vi "Read5160Record.vi"(11 "scope params":T1={"scope mode"=enum."Stopped", "ticker"=refnum, "record length"=0, "FPGA ref"=refnum, "P2P params"={"instrument handle"="", "stream session"=refnum, "scale"={"offset"=0.0, "gain"=0.0, "reserved 1"=0.0, "reserved 2"=0.0}, "actual sample rate"=10000000.0, "Trigger"=enum."PFI 0", "SCOPE Resource"="Dev1", "input impedance"=0}, "FPGA ref 5160"=refnum, "data mode"=enum."Real IO"} {"P2P params"."input impedance" items=["1 mega ohm"=0, "50 ohms"=2]; "P2P params"."actual sample rate" format="%.2p"}) -> (1 "Num elements":i32, 2 "data":i16[][](array[numeric]), 3 "scope params out":T1={"scope mode"=enum."Stopped", "ticker"=refnum, "record length"=0, "FPGA ref"=refnum, "P2P params"={"instrument handle"="", "stream session"=refnum, "scale"={"offset"=0.0, "gain"=0.0, "reserved 1"=0.0, "reserved 2"=0.0}, "actual sample rate"=10000000.0, "Trigger"=enum."PFI 0", "SCOPE Resource"="Dev1", "input impedance"=0}, "FPGA ref 5160"=refnum, "data mode"=enum."Real IO"} {"P2P params"."input impedance" items=["1 mega ohm"=0, "50 ohms"=2]; "P2P params"."actual sample rate" format="%.2p"}, 5 "P2P overflow":bool)   [LabVIEW 2013]
uses:
  controls/scope_params.ctl
  Utilities/Ticker/Ticker.lvclass
  controls/ScopeMode.ctl
  Config/FPGAref.ctl
  P2P params.ctl
  trigger_source.ctl
  Config/5160FPGAref.ctl
  FPGA/DataMode.ctl
  <vilib>/rvi/interface/common/niFpgaWaitOnOcc.vi
  <vilib>/Utility/error.llb/Error Cluster From Error Code.vi
  <vilib>/rvi/errors/niLvFpgaAdjustHostInterfaceError.vi
  <vilib>/rvi/interface/nirviReadWriteControl/nirviReadWriteControl.xnode
  <vilib>/rvi/interface/nirviMethod/nirviMethod.xnode
  <vilib>/FPGAPlugInAG/Dynamic/niLvFpga_ReadFifo_Dynamic.vi
  <vilib>/rvi/errors/niLvFpgaMergeErrorWithErrorCode.vi
  <resource>/objmgr/PeerToPeerStream.rc
  NiFpgaLv.dll
  <vilib>/rvi/interface/Simulation/niFpgaSimulationCallBeginRW.vi
panel:
  out "Data":u64[](array[numeric])
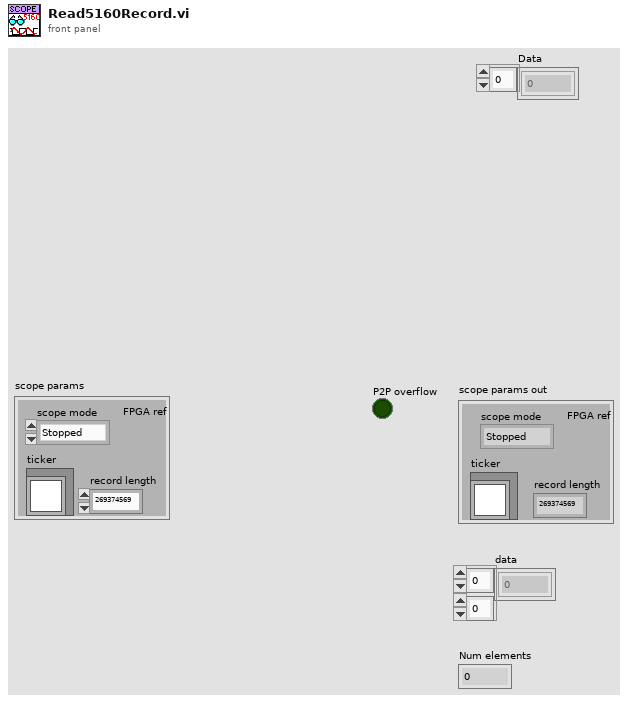
[diagram p1: front panel]
types:
  T1 = typedef "scope_params.ctl" = cluster{"scope mode":T2, "ticker":refnum<class "Ticker.lvclass">, "record length":u32, "FPGA ref":T3, "P2P params":T4, "FPGA ref 5160":T6, "data mode":T7}
  T2 = typedef "ScopeMode.ctl" = enum16{"Stopped", "Single", "Running"}
  T3 = typedef "FPGAref.ctl" = refnum<k20>
  T4 = typedef "P2P params.ctl" = cluster{"instrument handle":refnum<k15>, "stream session":refnum<k20>, "scale":cluster{"offset":dbl, "gain":dbl, "reserved 1":dbl, "reserved 2":dbl}, "actual sample rate":dbl, "Trigger":T5, "SCOPE Resource":refnum<k15>, "input impedance":u32}
  T5 = typedef "trigger_source.ctl" = enum16{"PFI 0", "PFI 1", "Software"}
  T6 = typedef "5160FPGAref.ctl" = refnum<k20>
  T7 = typedef "DataMode.ctl" = enum16{"Real IO", "Simulated"}
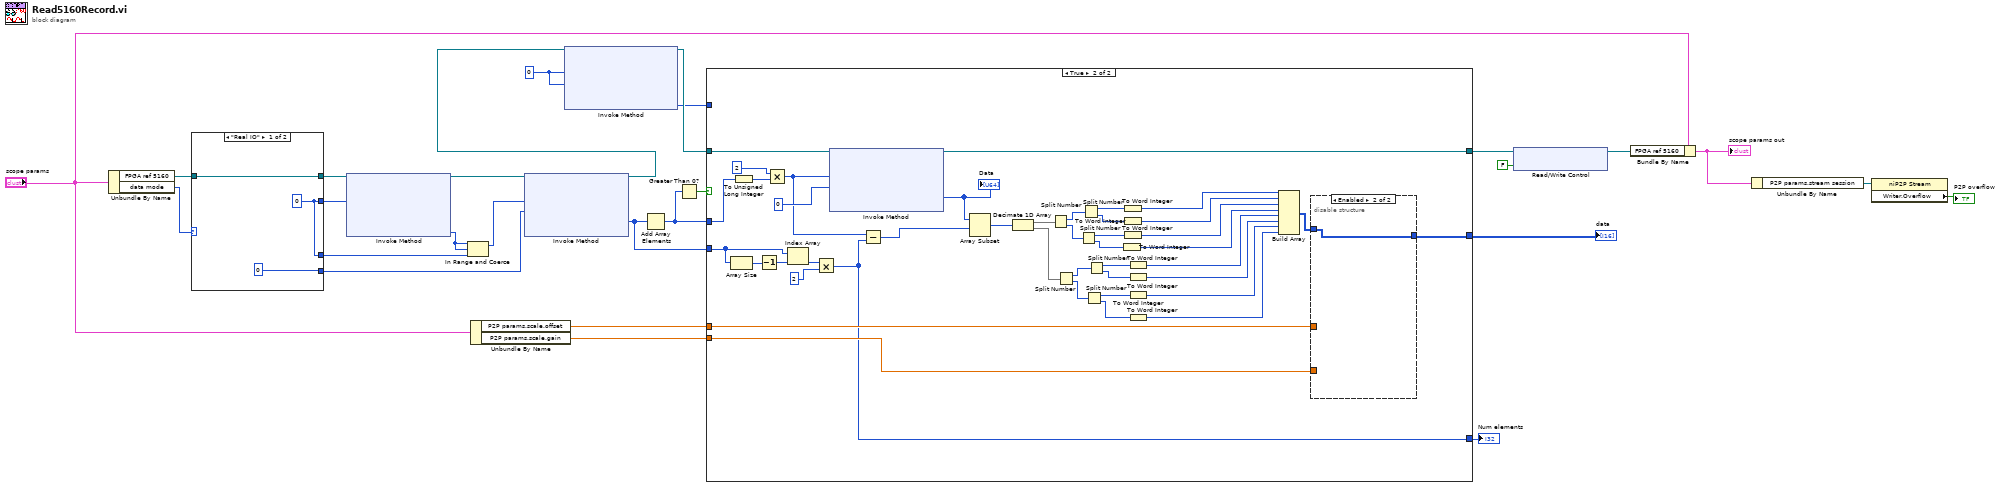
[diagram p0: block diagram]
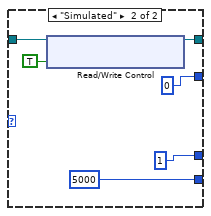
[diagram p2: hidden frame]
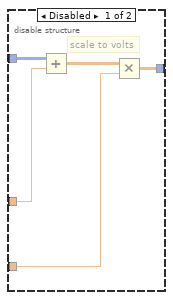
[diagram p4: hidden frame]
diagram:
  w7 = u32 0 ("Number of Elements")
  n1 = Unbundle By Name("scope params") -> ("FPGA ref 5160"=w14:T6, "data mode"=w15:T7)
  n2 = case shown="\"Real IO\"" w15 {
    tunnel: [0 ("Timeout (ms)") 5000 ("Timeout (ms)")] -> w4
    tunnel: w14 -> [w30 w36]
    tunnel: [w30 w34] -> w13
    tunnel: [w28 u32 0 ("Number of Elements")] -> w5
    tunnel: [w28 u32 1 ("Number of Elements")] -> w2
    frame "Real IO" {
      w28 = u32 0 ("Number of Elements")
    }
    frame "Simulated" {
      n3 = xnode "Read/Write Control"("FPGA VI Reference In"=w36, "Trigger simulated data"=TRUE) -> ("FPGA VI Reference Out"=w34:T6)  [unwired: 1 in, 1 out]
    }
  }
  n4 = xnode "Invoke Method"("FPGA VI Reference In"=w13, "Number of Elements"=w5) -> ("FPGA VI Reference Out"=w24:T6, "Elements Remaining"=w1:u32)  [unwired: 2 in, 2 out]
  n5 = In Range and Coerce(upper limit=w1, x=w1, lower limit=w2) -> (coerced(x)=w3:u32)  [unwired: 1 out]
  n6 = Unbundle By Name("scope params") -> ("P2P params.scale.offset"=w26:dbl, "P2P params.scale.gain"=w25:dbl)
  n7 = xnode "Invoke Method"("FPGA VI Reference In"=w24, "Number of Elements"=w3, "Timeout (ms)"=w4) -> ("FPGA VI Reference Out"=w9:T6, "Data"=w22:i32[])  [unwired: 1 in, 2 out]
  n8 = xnode "Invoke Method"("FPGA VI Reference In"=w9, "Number of Elements"=w7, "Timeout (ms)"=w7) -> ("FPGA VI Reference Out"=w8:T6, "Elements Remaining"=w6:u32)  [unwired: 1 in, 2 out]
  n9 = Add Array Elements(numeric array=w22) -> (sum=w23:i32)
  n10 = Greater Than 0?(x=w23) -> (x > 0?=w21:bool)
  n11 = case shown="True" w21 {
    tunnel: [_ w79] -> w27
    tunnel: w26 -> [_ w78]
    tunnel: w25 -> [_ w77]
    tunnel: w8 -> [w37 w53]
    tunnel: w23 -> [_ w45]
    tunnel: w22 -> [_ w52]
    tunnel: [w37 w51] -> w12
    tunnel: [_ w39] -> w20
    tunnel: w6 -> [_ _]
    frame False {
    }
    frame True {
      n12 = Array Size(array=w52) -> (size(s)=w49:i32)
      n13 = To Unsigned Long Integer(number=w45) -> (unsigned 32bit integer=w43:u32)
      n14 = Decrement(x=w49) -> (x-1=w48:i32)
      n15 = Multiply(x=u32 2, y=w43) -> (x*y=w38:u32)
      n16 = Index Array(array=w52, index=w48) -> (element=w41:i32)
      n17 = Multiply(x=w41, y=u32 2 ("x")) -> (x*y=w39:u32)
      n18 = xnode "Invoke Method"("FPGA VI Reference In"=w53, "Number of Elements"=w38, "Timeout (ms)"=0) -> ("FPGA VI Reference Out"=w51:T6, "Data"=w47:u64[])  [unwired: 1 in, 2 out]
      "Data" <- w47
      n19 = Subtract(x=w38, y=w39) -> (x-y=w46:u32)
      n20 = Array Subset(array=w47, index=w46) -> (w50:u64[])  [unwired: 1 in]
      n21 = Decimate 1D Array(w50) -> (w70:u64[], w59:u64[])
      n22 = Split Number(x=w70) -> (hi(x)=w72:u32[], lo(x)=w76:u32[])
      n23 = Split Number(x=w59) -> (hi(x)=w64:u32[], lo(x)=w60:u32[])
      n24 = Split Number(x=w76) -> (hi(x)=w74:u16[], lo(x)=w73:u16[])
      n25 = Split Number(x=w72) -> (hi(x)=w71:u16[], lo(x)=w75:u16[])
      n26 = Split Number(x=w60) -> (hi(x)=w62:u16[], lo(x)=w63:u16[])
      n27 = Split Number(x=w64) -> (hi(x)=w65:u16[], lo(x)=w61:u16[])
      n28 = To Word Integer(number=w73) -> (16bit integer=w66:i16[])
      n29 = To Word Integer(number=w71) -> (16bit integer=w69:i16[])
      n30 = To Word Integer(number=w75) -> (16bit integer=w68:i16[])
      n31 = To Word Integer(number=w74) -> (16bit integer=w67:i16[])
      n32 = To Word Integer(number=w65) -> (16bit integer=w58:i16[])
      n33 = To Word Integer(number=w61) -> (16bit integer=w57:i16[])
      n34 = To Word Integer(number=w62) -> (16bit integer=w56:i16[])
      n35 = To Word Integer(number=w63) -> (16bit integer=w55:i16[])
      n36 = Build Array(w69, w68, w67, w66, w58, w57, w56, w55) -> (w54:i16[][])
      n37 = disable-structure shown="Enabled" {
        disable-tunnel: [w84 w85] -> w79
        disable-tunnel: w78 -> [w83 _]
        disable-tunnel: w77 -> [w81 _]
        disable-tunnel: w54 -> [w80 w85]
        frame Disabled {
          # "scale to volts"
          n38 = Add(x=w80, y=w83) -> (x+y=w82:dbl[][])
          n39 = Multiply(x=w82, y=w81) -> (x*y=w84:dbl[][])
        }
        frame Enabled {
        }
      }
    }
  }
  "data" <- w27
  "Num elements" <- w20
  n40 = xnode "Read/Write Control"("FPGA VI Reference In"=w12, "Trigger simulated data"=FALSE) -> ("FPGA VI Reference Out"=w11:T6)  [unwired: 1 in, 1 out]
  n41 = Bundle By Name(cluster="scope params", "FPGA ref 5160"=w11) -> (w19:T1)
  "scope params out" <- w19
  n42 = Unbundle By Name(w19) -> ("P2P params.stream session"=w18:refnum<k20>)
  n43 = property class="niP2P Stream"(reference=w18) -> ("Writer.Overflow"=→"P2P overflow":bool)  [unwired: 1 in, 2 out]
